vi "Add Content Length.vi"(8 "error in (no error)":errorcluster, 10 "JSON Response String in":string) -> (0 "error out":errorcluster, 2 "JSON Response String out":string)   [LabVIEW 2020]
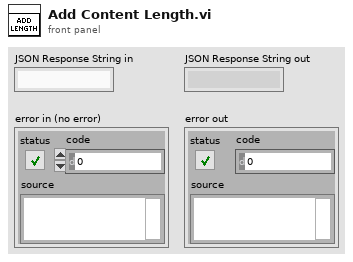
[diagram p1: front panel]
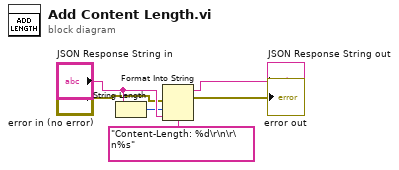
[diagram p0: block diagram]
diagram:
  n1 = String Length(string="JSON Response String in") -> (length=w1:i32)
  n2 = Format Into String(format string="Content-Length: %d\r\n\r\n%s", error in="error in (no error)", w1, "JSON Response String in") -> (resulting string=→"JSON Response String out":string, error out=→"error out":errorcluster)  [unwired: 1 in]
